vi "troca nome.vi"(1 "GO":refnum<vi>) -> (0 "acionou GO":bool)   [LabVIEW 2012]
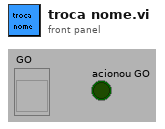
[diagram p1: front panel]
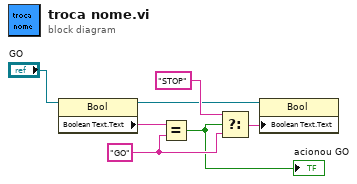
[diagram p0: block diagram]
diagram:
  w5 = "GO" ("Boolean Text.Text")
  n1 = property class="Bool"(reference="GO") -> (reference out=w3:refnum<vi>, "Boolean Text.Text"=w2:string)  [unwired: 1 in, 1 out]
  n2 = Equal?(x=w2, y=w5) -> (x = y?=w4:bool)
  "acionou GO" <- w4
  n3 = Select(t="STOP" ("Boolean Text.Text"), s=w4, f=w5) -> (s? t:f=w7:string)
  n4 = property class="Bool"(reference=w3, "Boolean Text.Text"=w7) -> ()  [unwired: 1 in, 2 out]
